vi "ULx Read (Composite 2D NChan NSamp).vi"(0 "task in":refnum<k24>, 7 "number of samples per channel":i32=-1, 9 "timeout":dbl=10.0 format="%_4g", 11 "error in":errorcluster) -> (4 "task out":refnum<k24>, 6 "analog data":dbl[][](array[numeric]), 8 "digital data":u32[][](array[numeric]) format="%#.0f", 10 "counter data":dbl[][](array[numeric]), 15 "error out":errorcluster)   [LabVIEW 2020]
doc: "Reads one or more samples from a task that contains one or more composite input channels."
uses:
  C:/Users/William/Documents/LV 2020 builds/LeaktestDAQ/Source-v33/ULx_LV.dll
  ULx_LV.dll
panel:
  # "channel"
  # "sample #"
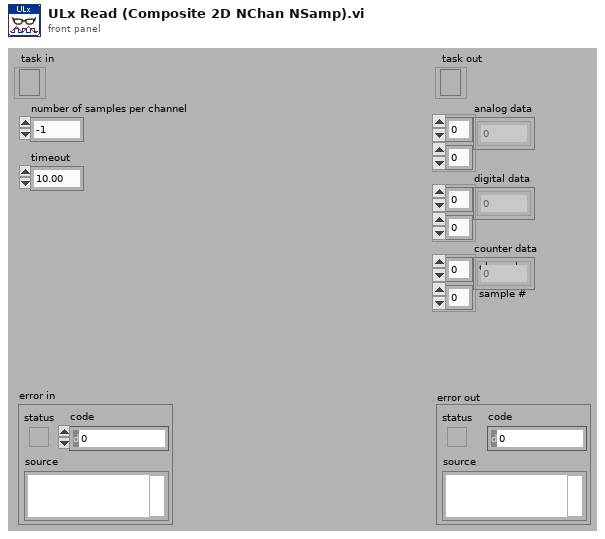
[diagram p1: front panel]
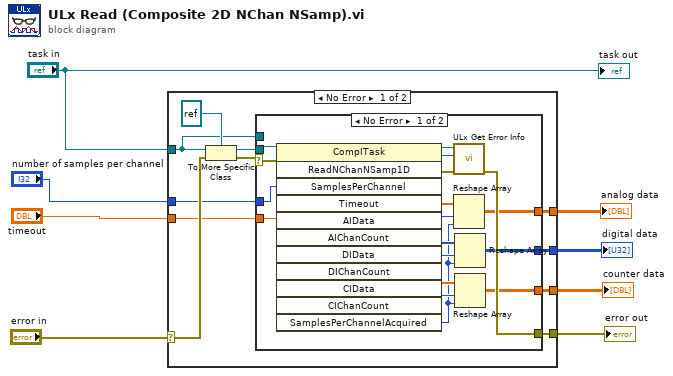
[diagram p0: block diagram]
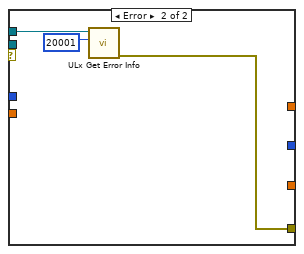
[diagram p2: hidden frame]
diagram:
  n1 = case shown="No Error" "error in" {
    selector: "error in" -> [w19 w41]
    tunnel: "task in" -> [w11 _]
    tunnel: "timeout" -> [w15 _]
    tunnel: [w12 _] -> w3
    tunnel: [w14 w41] -> w6
    tunnel: "number of samples per channel" -> [w13 _]
    tunnel: [w10 _] -> w2
    tunnel: [w9 _] -> w1
    frame No Error {
      n2 = To More Specific Class(target class=refnum<k24> refnum, reference=w11, error in=w19) -> (specific class reference=w16:refnum<k24>, error out=w17:errorcluster)
      n3 = case shown="No Error" w17 {
        selector: w17 -> [w36 _]
        tunnel: w16 -> [w37 _]
        tunnel: w15 -> [w32 _]
        tunnel: [w33 w38] -> w14
        tunnel: w13 -> [w31 _]
        tunnel: [w29 _] -> w12
        tunnel: w11 -> [_ w40]
        tunnel: [w24 _] -> w10
        tunnel: [w20 _] -> w9
        frame No Error {
          n4 = invoke class="CompITask" method="ReadNChanNSamp1D"(reference=w37, error in=w36, "SamplesPerChannel"=w31, "Timeout"=w32) -> (reference out=w34:refnum<k24>, error out=w35:errorcluster, "ReadNChanNSamp1D"=w30:i32, "AIData"=w28:dbl[], "AIChanCount"=w27:i32, "DIData"=w26:u32[], "DIChanCount"=w25:i32, "CIData"=w23:dbl[], "CIChanCount"=w22:i32, "SamplesPerChannelAcquired"=w21:i32)  [unwired: 8 in, 2 out]
          n5 = call "ULx Get Error Info.vi"("error in"=w35, "ErrorCode"=w30, "task in"=w34) -> ("error out"=w33:errorcluster)  [unwired: 8 in]
          n6 = Reshape Array(w28, w27, w21) -> (w29:dbl[][])
          n7 = Reshape Array(w26, w25, w21) -> (w24:u32[][])
          n8 = Reshape Array(w23, w22, w21) -> (w20:dbl[][])
        }
        frame Error {
          n9 = call "ULx Get Error Info.vi"("ErrorCode"=20001, "task in"=w40) -> ("error out"=w38:errorcluster)  [unwired: 9 in]
        }
      }
    }
    frame Error {
    }
  }
  "error out" <- w6
  "analog data" <- w3
  "digital data" <- w2
  "counter data" <- w1
  "task out" <- "task in"
